vi "dfd_FXP PtByPt Lattice Allpass (basic).vi"(6 "state in":i64[](array[numeric]), 7 "FXPOPs":T5[](array[typedef]) {"source" items=["Coef a/k"=0, "Coef b/v"=7, "Input"=1, "Output"=2, "Multiplicand"=3, "Product"=4, "Sum"=5, "Delay"=6, "Gain"=8]}, 8 "filtering statistics in":T4(array[cluster]) {"statistics information"."min value" format="%.2f"; "statistics information"."max value" format="%.2f"; "Quantizer Source" items=["Coefficients a/k"=0, "Coefficients b/v"=7, "Input"=1, "Output"=2, "Multiplicand"=3, "Product"=4, "Sum"=5, "Delay"=6]}, 10 "coef k[M..1]":T1, 11 "x":T7={"value"=0, "wl"=0, "iwl"=0, "Signed"=TRUE} {"value" format="%.0x"}) -> (0 "filtering statistics out":T4(array[cluster]) {"statistics information"."min value" format="%.2f"; "statistics information"."max value" format="%.2f"; "Quantizer Source" items=["Coefficients a/k"=0, "Coefficients b/v"=7, "Input"=1, "Output"=2, "Multiplicand"=3, "Product"=4, "Sum"=5, "Delay"=6]}, 3 "filtered x":T7={"value"=0, "wl"=0, "iwl"=0, "Signed"=TRUE} {"value" format="%.0x"}, 4 "state out":i64[](array[numeric]))   [LabVIEW 2017, in "NI_DigFilter_FXP.lvlib"]
uses:
  <vilib>/addons/Digital Filter Design/NI_DigFilter_FXP.lvlib
  <vilib>/addons/Digital Filter Design/_Objects.llb/dfd_DFXP Data Type (scaler).ctl
  <vilib>/addons/Digital Filter Design/_Objects.llb/dfd_DFXP Operation Parameter.ctl
  <vilib>/addons/Digital Filter Design/_Objects.llb/dfd_Internal Quantization Srcs.ctl
  <vilib>/addons/Digital Filter Design/_Objects.llb/dfd_DFXP Data Type (vector).ctl
  <vilib>/addons/Digital Filter Design/_Objects.llb/DFD Quantization Sources.ctl
  <vilib>/addons/Digital Filter Design/_Objects.llb/DFD FXP Statistics Data.ctl
  <vilib>/addons/Digital Filter Design/NI_DigFilterLicensed.lvlib
panel:
  in  "DFXP array type":T1
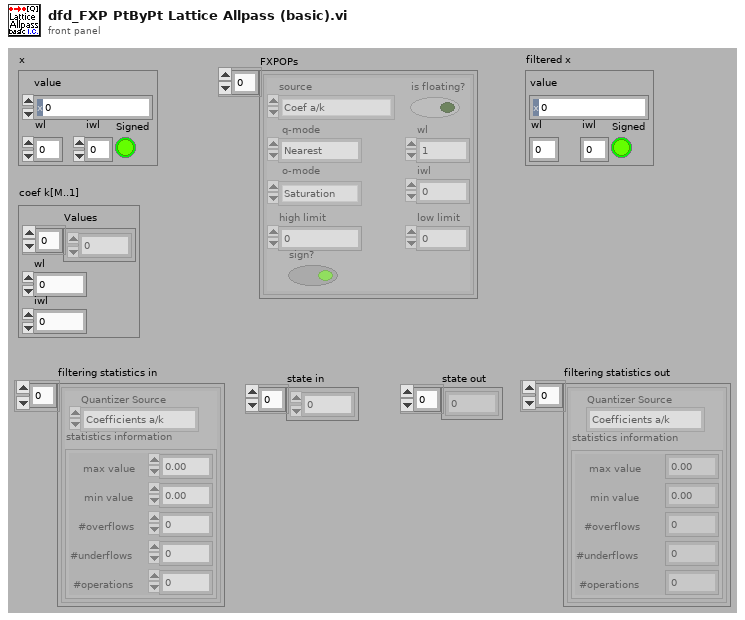
[diagram p1: front panel]
types:
  T1 = typedef "dfd_DFXP Data Type (vector).ctl" = cluster{"Values":i64[], "wl":i16, "iwl":i16}
  T2 = typedef "NI_DigFilterLicensed.lvlib/DFD Quantization Sources.ctl" = u16
  T3 = typedef "NI_DigFilterLicensed.lvlib/DFD FXP Statistics Data.ctl" = cluster{"max value":ext, "min value":ext, "#overflows":i32, "#underflows":i32, "#operations":i32}
  T4 = cluster{"Quantizer Source":T2, "statistics information":T3}[]
  T5 = typedef "dfd_DFXP Operation Parameter.ctl" = cluster{"source":T6, "is floating?":bool, "o-mode":enum16{"Saturation", "Wrap"}, "q-mode":enum16{"Nearest", "Truncation"}, "wl":i16, "high limit":i64, "low limit":i64, "iwl":i16, "sign?":bool}
  T6 = typedef "NI_DigFilterLicensed.lvlib/dfd_Internal Quantization Srcs.ctl" = u16
  T7 = typedef "dfd_DFXP Data Type (scaler).ctl" = cluster{"value":i64, "wl":i16, "iwl":i16, "Signed":bool}
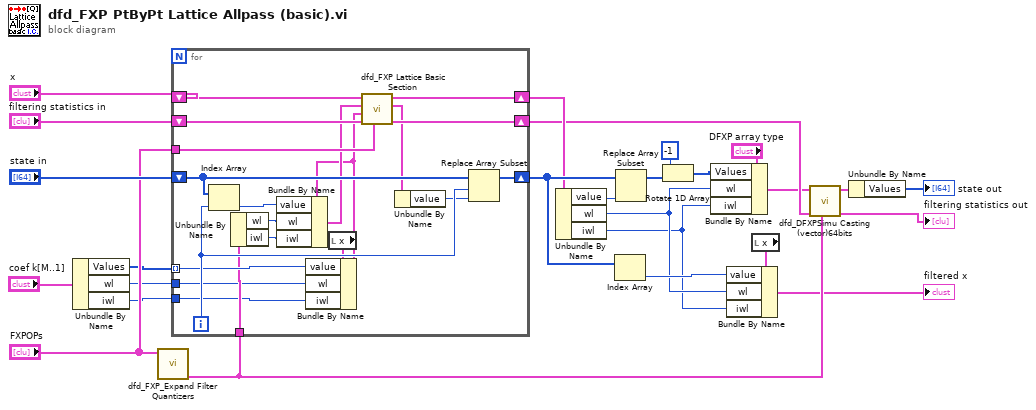
[diagram p0: block diagram]
diagram:
  n1 = Unbundle By Name("coef k[M..1]") -> ("Values"=w3:i64[], "wl"=w2:i16, "iwl"=w1:i16)
  n2 = call <vilib>:"dfd_FXP_Expand Filter Quantizers.vi"("FXPOPs"="FXPOPs") -> ("Delay"=w12:T5)  [unwired: 10 out]
  n3 = for {
    shift-right: [w42] -> w20
    shift-left: "x" -> [w43]
    shift-right: [w45] -> w21
    shift-left: "state in" -> [w46]
    tunnel: "FXPOPs" -> [w41]
    shift-right: [w38] -> w15
    shift-left: "filtering statistics in" -> [w40]
    tunnel: w3 -> [w36] mode=indexing
    tunnel: w12 -> [w32]
    tunnel: w2 -> [w28]
    tunnel: w1 -> [w27]
    i -> [w44]
    n4 = Index Array(array=w46, index=w44) -> (element=w39:i64)
    n5 = Unbundle By Name(w32) -> ("wl"=w31:i16, "iwl"=w30:i16)
    n6 = local read "x"() -> (w35:T7)
    n7 = Bundle By Name(cluster=w35, "value"=w36, "wl"=w28, "iwl"=w27) -> (w33:T7)
    n8 = Bundle By Name(cluster=w33, "value"=w39, "wl"=w31, "iwl"=w30) -> (w34:T7)
    n9 = call <vilib>:"dfd_FXP Lattice Basic Section.vi"("FXPOPs"=w41, "filtering statistics in"=w40, "k(m)"=w33, "w(m-1)"=w34, "x(m)"=w43) -> ("filtering statistics out"=w38:T4, "w(m)"=w37:T7, "x(m-1)"=w42:T7)  [unwired: 1 out]
    n10 = Unbundle By Name(w37) -> ("value"=w29:i64)
    n11 = Replace Array Subset(array=w46, new element=w29, index=w44) -> (w45:i64[])
  }
  n12 = Unbundle By Name(w20) -> ("value"=w11:i64, "wl"=w6:i16, "iwl"=w5:i16)
  n13 = Index Array(array=w21) -> (element=w16:i64)  [unwired: 1 in]
  n14 = Replace Array Subset(array=w21, new element=w11) -> (w26:i64[])  [unwired: 1 in]
  n15 = Rotate 1D Array(1:w26, 2:-1 ("n")) -> (0:w18:i64[])
  n16 = Bundle By Name(cluster="DFXP array type", "Values"=w18, "wl"=w6, "iwl"=w5) -> (w8:T1)
  n17 = local read "x"() -> (w7:T7)
  n18 = Bundle By Name(cluster=w7, "value"=w16, "wl"=w6, "iwl"=w5) -> (→"filtered x":T7)
  n19 = call <vilib>:"dfd_DFXPSimu Casting (vector)64bits.vi"("op params"=w12, "filtering statistics in"=w15, "Value in"=w8) -> ("filtering statistics out"=→"filtering statistics out":T4, "Value out"=w17:T1)  [unwired: 1 in, 6 out]
  n20 = Unbundle By Name(w17) -> ("Values"=→"state out":i64[])
